vi "SetSerializableDataCommon.vi"(7 "BlueSerializer in":refnum<class "BlueSerializer.lvclass">, 8 "error in (no error)":errorcluster, 10 "Data In":T1={"StructuredData"=variant(string ""), "ClassOps (child, parent)"=[]}, 11 "SerializableData":variant) -> (0 "error out":errorcluster, 2 "Data Out":T1={"StructuredData"=variant(string ""), "ClassOps (child, parent)"=[]}, 3 "SerializableData":variant, 5 "BlueSerializer out":refnum<class "BlueSerializer.lvclass">)   [LabVIEW 2019, in "BlueSerialization.lvlib" / "BlueSerializer.lvclass"]
uses:
  BlueSerializer.lvclass
  SetSerializableDataCluster.ctl
  SetSerializableDataClusterIterable.ctl
  BlueSerializable/BlueSerializable.lvclass
  SetSerializableDataClusterLayer.ctl
  BlueSerializableVersion.ctl
  SetSerializableDataObject.ctl
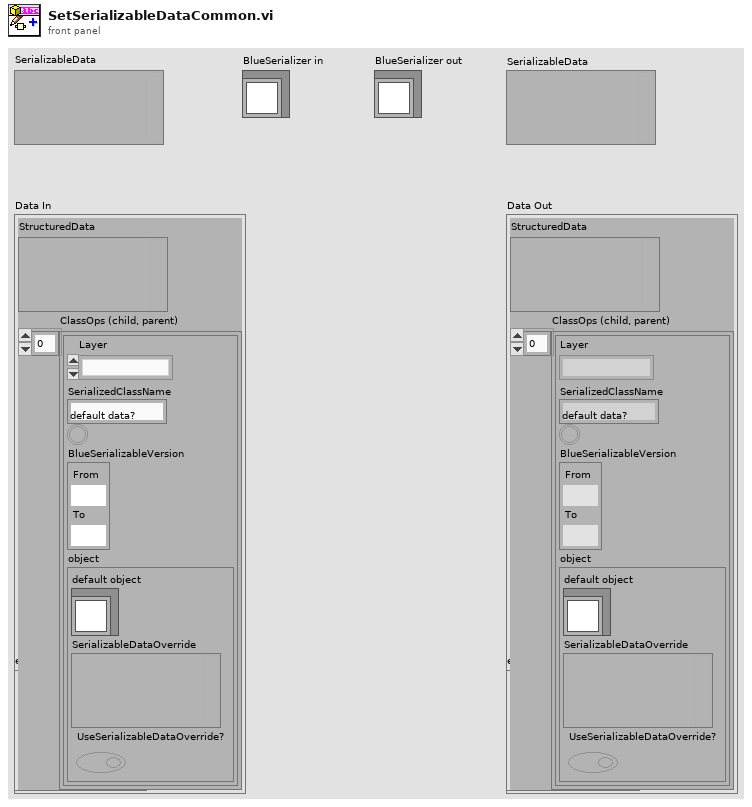
[diagram p1: front panel]
types:
  T1 = typedef "BlueSerialization.lvlib/BlueSerializer.lvclass/SetSerializableDataCluster.ctl" = cluster{"StructuredData":variant, "ClassOps (child, parent)":T2[]}
  T2 = typedef "BlueSerialization.lvlib/BlueSerializer.lvclass/SetSerializableDataClusterIterable.ctl" = cluster{"Layer":T3, "SerializedClassName":string, "default data?":bool, "BlueSerializableVersion":T4, "object":T5}
  T3 = typedef "BlueSerialization.lvlib/BlueSerializer.lvclass/SetSerializableDataClusterLayer.ctl" = enum16{"new class layer", "dropped class layer", "agreed class layer"}
  T4 = typedef "BlueSerialization.lvlib/BlueSerializer.lvclass/BlueSerializableVersion.ctl" = cluster{"From":u16, "To":u16}
  T5 = typedef "BlueSerialization.lvlib/BlueSerializer.lvclass/SetSerializableDataObject.ctl" = cluster{"default object":refnum<class "BlueSerializable.lvclass">, "SerializableDataOverride":variant, "UseSerializableDataOverride?":bool}
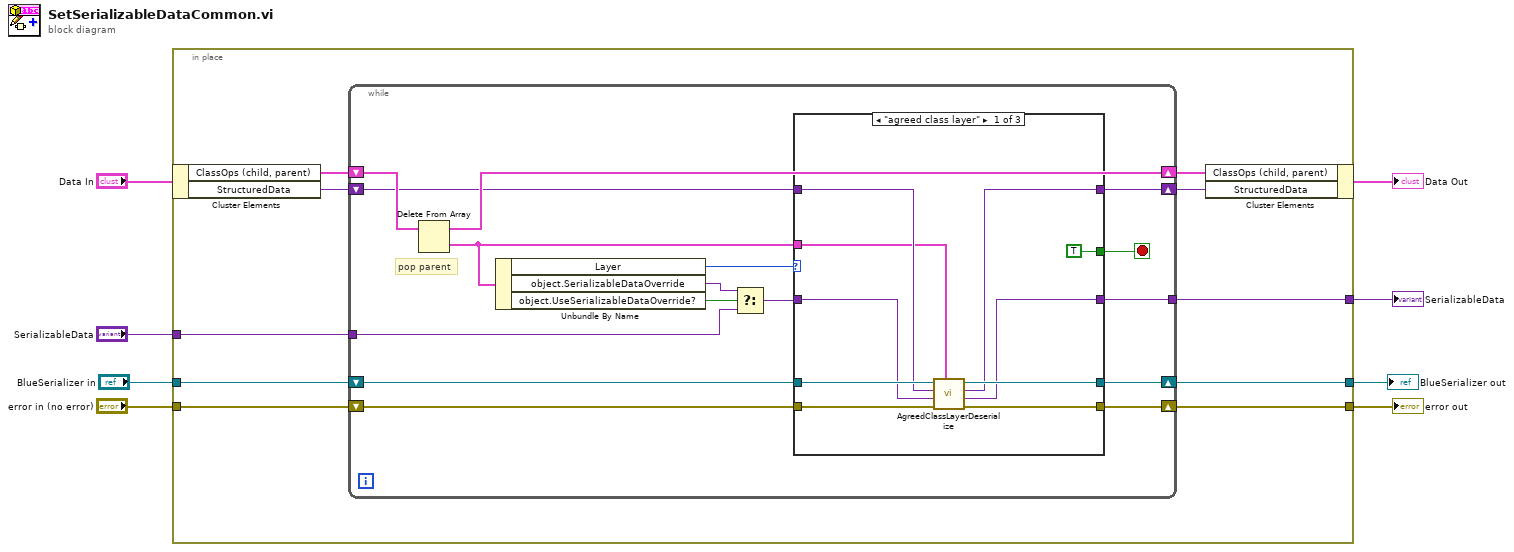
[diagram p0: block diagram]
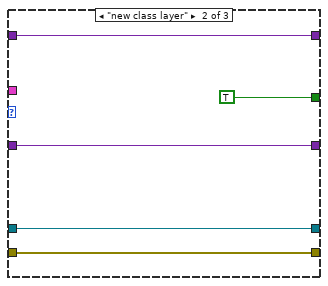
[diagram p2: hidden frame]
diagram:
  n1 = in-place {
    in-place-border: "error in (no error)" -> [w16]
    in-place-border: [w12] -> w5
    in-place-border: "SerializableData" -> [w10]
    in-place-border: [w9] -> w4
    in-place-border: "BlueSerializer in" -> [w15]
    in-place-border: [w13] -> w1
    n2 = in-place-cluster #1("Data In") -> ("ClassOps (child, parent)"=w18:T2[], "StructuredData"=w14:variant)
    n3 = while {
      shift-right: [w33] -> w17
      shift-left: w18 -> [w34]
      shift-right: [w28] -> w12
      shift-left: w16 -> [w32]
      shift-right: [w29] -> w13
      shift-left: w15 -> [w31]
      shift-right: [w27] -> w11
      shift-left: w14 -> [w30]
      tunnel: w10 -> [w20]
      tunnel: [w24] -> w9
      stop <- w25 stop-if-true
      # "pop parent"
      n4 = Delete From Array(array=w34) -> (deleted portion=w23:T2, array with subset deleted=w33:T2[])  [unwired: 2 in]
      n5 = Unbundle By Name(w23) -> ("Layer"=w26:T3, "object.SerializableDataOverride"=w21:variant, "object.UseSerializableDataOverride?"=w22:bool)
      n6 = Select(t=w21, s=w22, f=w20) -> (s? t:f=w19:variant)
      n7 = case shown="\"agreed class layer\"" w26 {
        tunnel: w32 -> [w42 w45 w50]
        tunnel: w31 -> [w43 w46 w51]
        tunnel: w30 -> [w38 w49 w52]
        tunnel: w19 -> [w36 w47 _]
        tunnel: [w41 w46 w51] -> w29
        tunnel: [w37 w47 _] -> w24
        tunnel: [w40 w45 w50] -> w28
        tunnel: [w39 w49 w52] -> w27
        tunnel: [TRUE TRUE _] -> w25
        tunnel: w23 -> [w35 _ _]
        frame "agreed class layer" {
          n8 = call "AgreedClassLayerDeserialize.vi"("ClassOp"=w35, "error in (no error)"=w42, "SerializableData"=w36, "StructuredData"=w38, "BlueSerializer in"=w43) -> ("error out"=w40:errorcluster, "Variant"=w37:variant, "StructuredData"=w39:variant, "BlueSerializer out"=w41:refnum<class "BlueSerializer.lvclass">)  [unwired: 3 in]
        }
        frame "new class layer" {
        }
        frame "dropped class layer" {
        }
      }
    }
    n9 = in-place-cluster #1("ClassOps (child, parent)"=w17, "StructuredData"=w11) -> (→"Data Out":T1)
  }
  "error out" <- w5
  "SerializableData" <- w4
  "BlueSerializer out" <- w1
